vi "Increment Iteration.vi"(8 "error in (no error)":errorcluster, 11 "Framework State in":refnum<class "Framework State.lvclass">) -> (0 "error out":errorcluster, 3 "Framework State out":refnum<class "Framework State.lvclass">)   [LabVIEW 2017, in "DSF Core.lvlib" / "Framework State.lvclass"]
uses:
  Framework State.lvclass
  Framework State.lvclass/Framework State.ctl
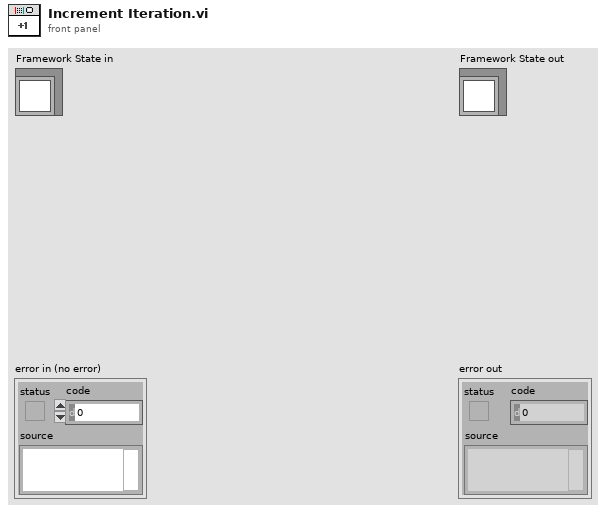
[diagram p1: front panel]
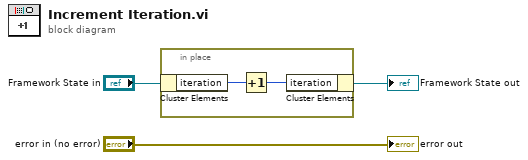
[diagram p0: block diagram]
diagram:
  n1 = in-place {
    n2 = in-place-cluster #1("Framework State in") -> ("iteration"=w5:u64)
    n3 = Increment(x=w5) -> (x+1=w4:u64)
    n4 = in-place-cluster #1("iteration"=w4) -> (→"Framework State out":refnum<class "Framework State.lvclass">)
  }
  "error out" <- "error in (no error)"
